vi "Get Models (OpenAI).vi"(8 "error in (no error)":errorcluster, 10 "url":string, 11 "Refnum in":T1) -> (0 "error out":errorcluster, 1 "Available Models":string[](array[string]), 2 "body":string, 3 "Refnum out":T1)   [LabVIEW 2023, in "LabVIEW LLM.lvlib"]
uses:
  LabVIEW LLM.lvlib
  <vilib>/httpClient/ClientHandle.ctl
  <vilib>/httpClient/LabVIEWHTTPClient.lvlib
  labview-ai-share/LabVIEW AI Base.lvlib
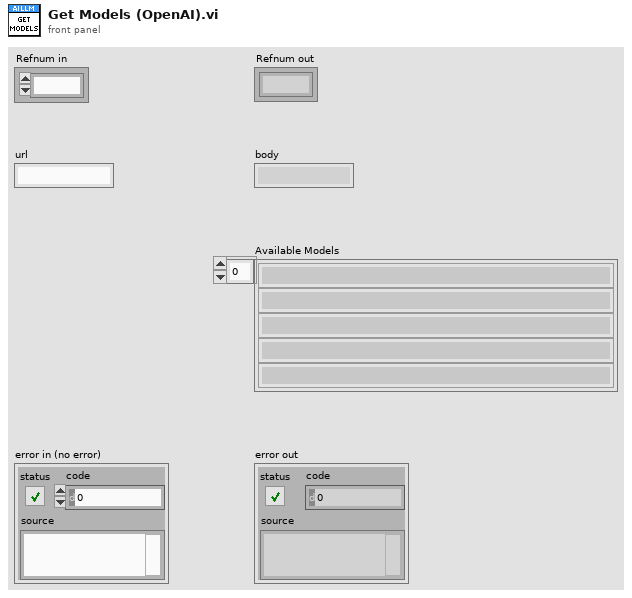
[diagram p1: front panel]
types:
  T1 = typedef "LabVIEWHTTPClient.lvlib/ClientHandle.ctl" = refnum<k1>
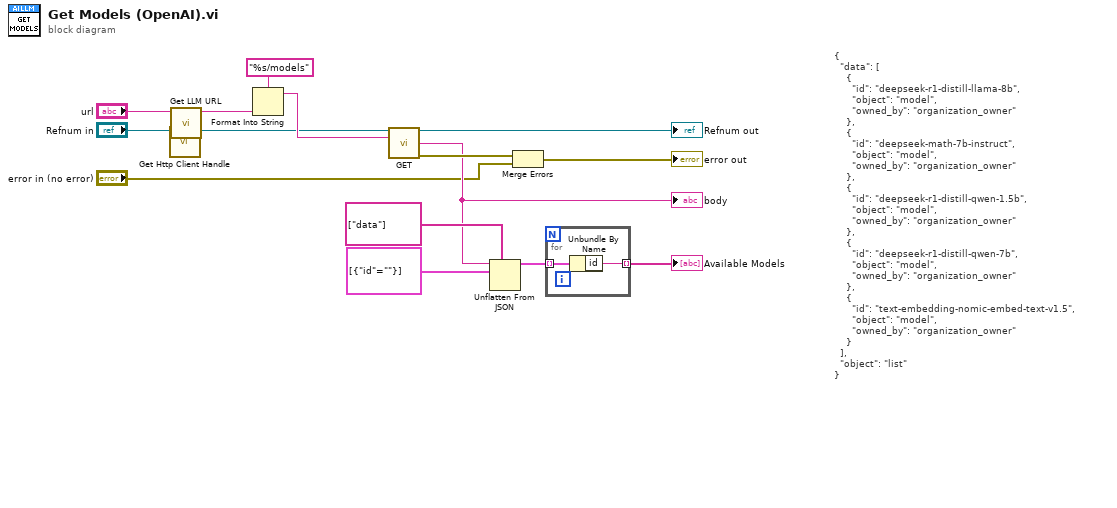
[diagram p0: block diagram]
diagram:
  # "{\n  \"data\": [\n    {\n      \"id\": \"deepseek-r1-distill-llama-8b\",\n      \"object\": \"model\",\n      \"owned_by\": \"organization_owner\"\n    },\n    {\n      \"id\": \"deepseek-math-7b-instruct\",\n      \"object\": \"model\",\n      \"owned_by\": \"organization_owner\"\n    },\n    {\n      \"id\": \"deepseek-r1-distill-qwen-1.5b\",\n      \"object\": \"model\",\n      \"owned_by\": \"organization_owner\"\n    },\n    {\n      \"id\": \"deepseek-r1-distill-qwen-7b\",\n      \"object\": \"model\",\n      \"owned_by\": \"organization_owner\"\n    },\n    {\n      \"id\": \"text-embedding-nomic-embed-text-v1.5\",\n      \"object\": \"model\",\n      \"owned_by\": \"organization_owner\"\n    }\n  ],\n  \"object\": \"list\"\n}"
  n1 = call "Get Http Client Handle.vi"("Refnum in"="Refnum in") -> ("Refnum out"=w1:T1)  [unwired: 10 in]
  n2 = call "Get LLM URL.vi"("OpenAI API URL"="url") -> ("OpenAI API URL"=w2:string)  [unwired: 10 in]
  n3 = Format Into String(format string="%s/models" ("url"), w2) -> (resulting string=w14:string)  [unwired: 2 in, 1 out]
  n4 = call <vilib>:"GET.vi"("client handle"=w1, "url"=w14) -> ("client handle out"=→"Refnum out":T1, "body"=w7:string, "error out"=w12:errorcluster)  [unwired: 10 in, 1 out]
  "body" <- w7
  n5 = Unflatten From JSON(path=string[] ["data"], JSON string=w7, type and defaults=cluster{"id":string}[] [{"id"=""}] ("path")) -> (value=w6:cluster{"id":string}[])  [unwired: 4 in, 1 out]
  n6 = Merge Errors(w12, "error in (no error)") -> (→"error out":errorcluster)
  n7 = for {
    tunnel: w6 -> [w17] mode=indexing
    tunnel: [w16] -> w5 mode=indexing
    n8 = Unbundle By Name(w17) -> ("id"=w16:string)
  }
  "Available Models" <- w5
